vi "GEOM_SortROIs.vi"(10 "ROIs":T2) -> (1 "Extreme Coords":T1={"xstart"=1, "ystart"=1, "xsize"=1, "ysize"=1})   [LabVIEW 2016]
uses:
  GEOM_ROI.ctl
  GEOM_Coords.ctl
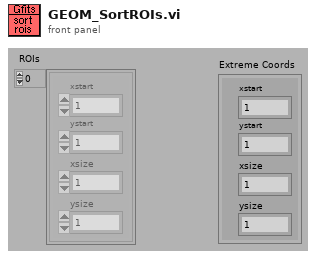
[diagram p1: front panel]
types:
  T1 = typedef "GEOM_Coords.ctl" = cluster{"xstart":u32, "ystart":u32, "xsize":u32, "ysize":u32}
  T2 = typedef "GEOM_ROI.ctl" = T1[]
  T3 = cluster{"xstart":i32, "ystart":i32, "xend":i32, "yend":i32}
  T4 = cluster{"xstart":i32, "ystart":i32, "xsize":i32, "ysize":i32}
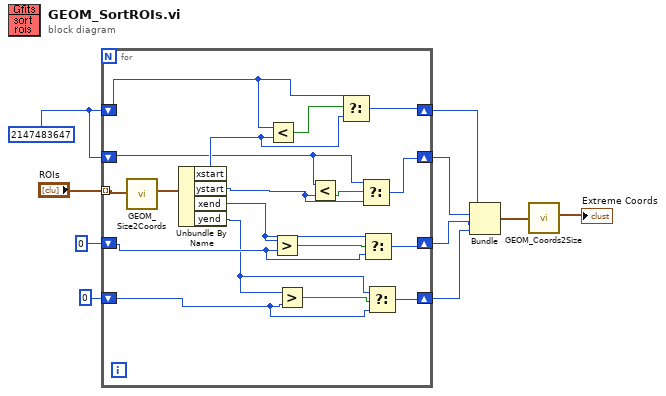
[diagram p0: block diagram]
diagram:
  w9 = 2147483647
  n1 = for {
    tunnel: "ROIs" -> [w28] mode=indexing
    shift-right: [w23] -> w6
    shift-left: w9 -> [w25]
    shift-right: [w19] -> w5
    shift-left: w9 -> [w21]
    shift-right: [w15] -> w4
    shift-left: 0 -> [w16]
    shift-right: [w11] -> w3
    shift-left: 0 -> [w12]
    n2 = call "GEOM_Size2Coords.vi"("Size"=w28) -> ("Coords"=w27:T3)  [unwired: 10 out]
    n3 = Unbundle By Name(w27) -> ("xstart"=w24:i32, "ystart"=w20:i32, "xend"=w17:i32, "yend"=w14:i32)
    n4 = Less?(x=w25, y=w24) -> (x < y?=w26:bool)
    n5 = Greater?(x=w17, y=w16) -> (0:w18:bool)
    n6 = Greater?(x=w14, y=w12) -> (0:w13:bool)
    n7 = Less?(x=w21, y=w20) -> (x < y?=w22:bool)
    n8 = Select(t=w25, s=w26, f=w24) -> (s? t:f=w23:i32)
    n9 = Select(t=w21, s=w22, f=w20) -> (s? t:f=w19:i32)
    n10 = Select(t=w17, s=w18, f=w16) -> (s? t:f=w15:i32)
    n11 = Select(t=w14, s=w13, f=w12) -> (s? t:f=w11:i32)
  }
  n12 = Bundle(w6, w5, w4, w3) -> (w2:cluster{i32, i32, i32, i32})  [unwired: 1 out]
  n13 = call "GEOM_Coords2Size.vi"("Coords"=w2) -> ("Size"=→"Extreme Coords":T4)  [unwired: 10 out]
